vi "Configure Parent Class.vi"(8 "error in (no error)":errorcluster, 10 "Parent Class":string, 11 "New Class Dialog In":refnum<class "New Class Dialog.lvclass">) -> (0 "error out":errorcluster, 3 "New Class Dialog Out":refnum<class "New Class Dialog.lvclass">)   [LabVIEW 2020, in "Process Generation.lvlib" / "New Class Dialog.lvclass"]
uses:
  New Class Dialog.lvclass
  New Class Dialog.lvclass/New Class Dialog.ctl
  Process Generator/Process Generator.lvclass
  Framework/Process/Process.lvclass
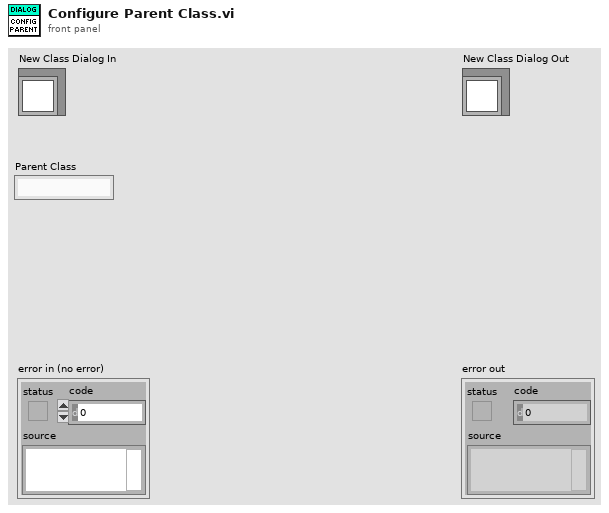
[diagram p1: front panel]
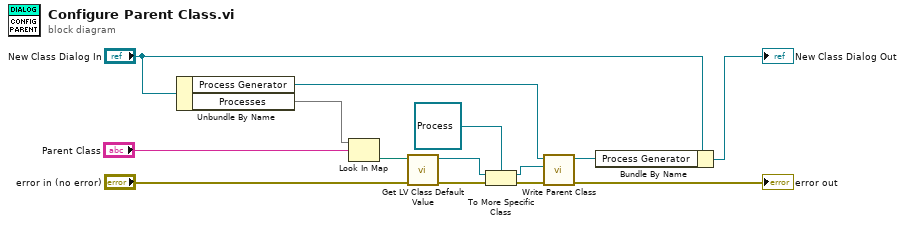
[diagram p0: block diagram]
diagram:
  n1 = Unbundle By Name("New Class Dialog In") -> ("Process Generator"=w6:refnum<class "Process Generator.lvclass">, "Processes"=w14:map{string, path})
  n2 = Look In Map(map=w14, key="Parent Class") -> (value=w3:path)  [unwired: 1 in, 1 out]
  n3 = call <vilib>:"Get LV Class Default Value.vi"("error in (no error)"="error in (no error)", "class path"=w3) -> ("error out"=w8:errorcluster, "object"=w10:refnum<class>)  [unwired: 8 in]
  n4 = To More Specific Class(target class=refnum<class "Process.lvclass"> refnum ("Parent Process"), reference=w10, error in=w8) -> (specific class reference=w12:refnum<class "Process.lvclass">, error out=w7:errorcluster)
  n5 = call "Write Parent Class.vi"("error in (no error)"=w7, "Parent Process"=w12, "Process Generator in"=w6) -> ("error out"=→"error out":errorcluster, "Process Generator out"=w1:refnum<class "Process Generator.lvclass">)  [unwired: 7 in]
  n6 = Bundle By Name(cluster="New Class Dialog In", "Process Generator"=w1) -> (→"New Class Dialog Out":refnum<class "New Class Dialog.lvclass">)
